vi "DEI_7420_TCP.vi"() -> ()   [LabVIEW 2012]
panel:
  in  "power on exit":bool
  in  "FORCE EXIT":bool
  out "Output Warning":bool
  in  "DEI Current Pulsar":enum32{"Control and Status"}(tab)
  in  "Amp On/Off":bool
  in  "INT TRIG FREQ":i32=7000 min=1000 max=100000 step=1000
  in  "MAIN PULSEWIDTH msec":dbl=1.0 min=0.05 max=5000.0 step=0.001 format="%.3g"
  in  "BIAS PULSEWIDTH msec":dbl=0.025 min=0.0 max=25000.0 step=0.001 format="%.3f"
  in  "BIAS CURRENT (A)":dbl min=0.0 max=5.8 step=0.001 format="%.3f"
  in  "MAIN CURRENT (A)":dbl=10.0 min=0.0 max=15.7 step=0.001 format="%.3g"
  in  "TRIGGER SOURCE":u16(ring)=1 items=["Internal", "External"]
  in  "EXT TRIG TERM (Ohms)":i32=50 min=50 max=10000 step=1
  in  "IP address":string="192.168.0.200"
  out "Int Trig Freq":string
  out "Main Current":string
  out "Main Pulsewidth":string
  out "Bias Current":string
  out "Bias Pulsewidth":string
  out "Ext Trig Term":string
  out "Trigger":string
  in  "Enable Output":bool
  in  "Set Values":bool
  out "Temp Out (C)":dbl
  out "Temp In (C)":dbl
  out "Rear Enable":bool
  out "Keyswitch Enable":bool
  in  "IP timeout ms":i32=1000
  out "Loop Count":i32=13
  in  "EXIT":bool
  # "DEI 7420 Current Pulsar"
  # "DEI\nRESPONSE"
  # "DEI\nCONTROLS"
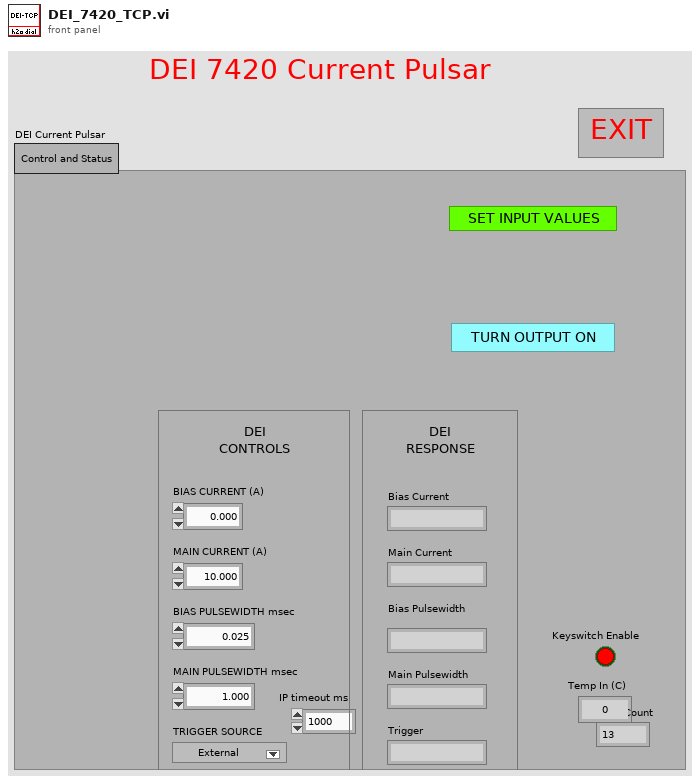
[diagram p1: front panel]
types:
  T1 = enum16{"*IDN?", "BIAS:CURRENT:SETPOINT?", "BIAS:CURRENT:SETPOINT", "FAULT?", "FAULT:CLEAR:ALL", "MAIN:CURRENT:SETPOINT?", "MAIN:CURRENT:SETPOINT", "OUTPUT?", "OUTPUT:DISABLE", "OUTPUT:ENABLE", "*RECALL", "*SAVE", "STATUS:KEYSWITCH?", "STATUS:REAR:ENABLE?", "TEMP:EXHAUST?", "TEMP:IN?", "TRIG?", "TRIG:EXTERNAL", "TRIG:INTERNAL", "TRIG:EXT:TERM?", "TRIG:EXT:TERM", "TRIG:INT:FREQ?", "TRIG:INT:FREQ", "TRIG:INT:BIAS:PULSEWIDTH?", "TRIG:INT:BIAS:PULSEWIDTH", "TRIG:INT:MAIN:PULSEWIDTH?", "TRIG:INT:MAIN:PULSEWIDTH"}
  T2 = enum16{"*IDN?", "BIAS:CURRENT:SETPOINT?", "BIAS:CURRENT:SETPOINT", "FAULT?", "FAULT:CLEAR:ALL", "MAIN:CURRENT:SETPOINT?", "MAIN:CURRENT:SETPOINT", "OUTPUT?", "OUTPUT:DISABLE", "OUTPUT:ENABLE", "*RECALL", "*SAVE", "STATUS:KEYSWITCH?", "STATUS:REAR:ENABLE?", "TEMP:EXHAUST?", "TEMP:IN?", "TRIG?", "TRIG:EXTERNAL", "TRIG:INTERNAL", "TRIG:EXT:TERM?", "TRIG:EXT:TERM", "TRIG:INT:FREQ?", "TRIG:INT:FREQ", "TRIG:INT:BIAS:PULSEWIDTH?", "TRIG:INT:BIAS:PULSEWIDTH", "TRIG:INT:MAIN:PULSEWIDTH?", "TRIG:INT:MAIN:PULSEWIDTH"}[]
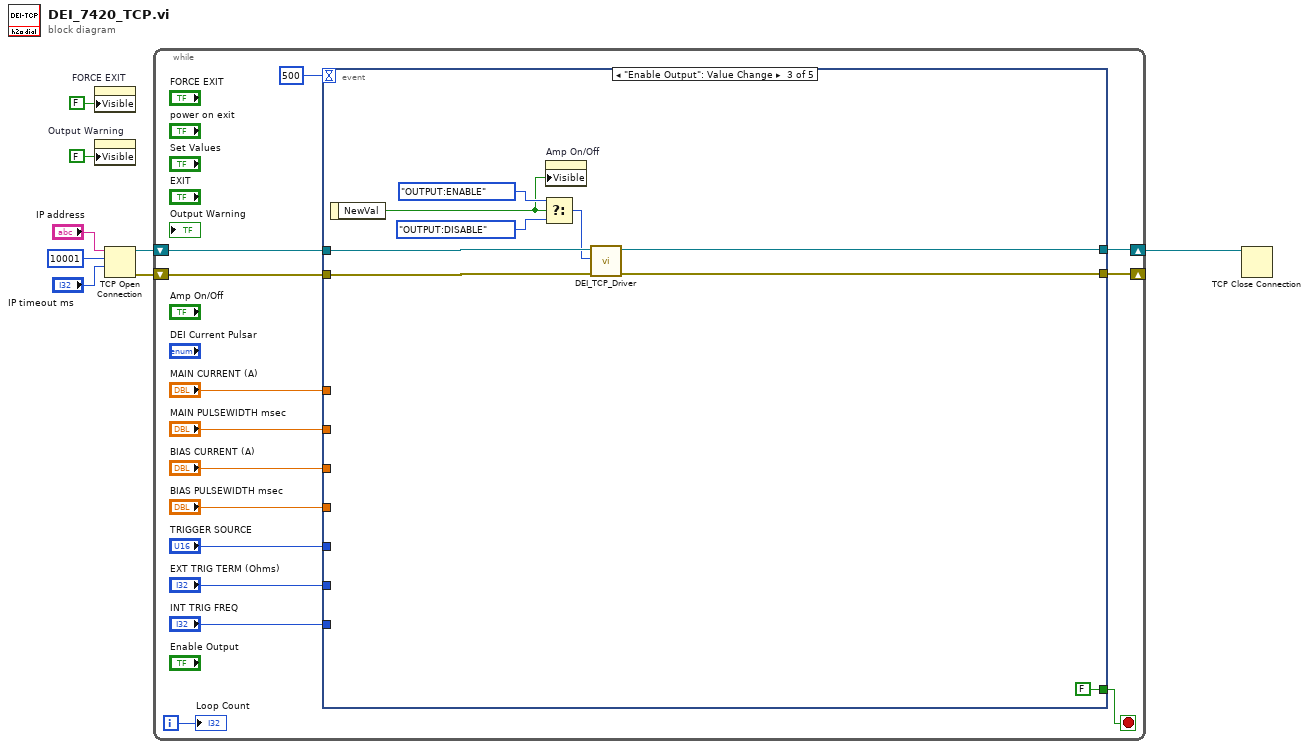
[diagram p0: block diagram]
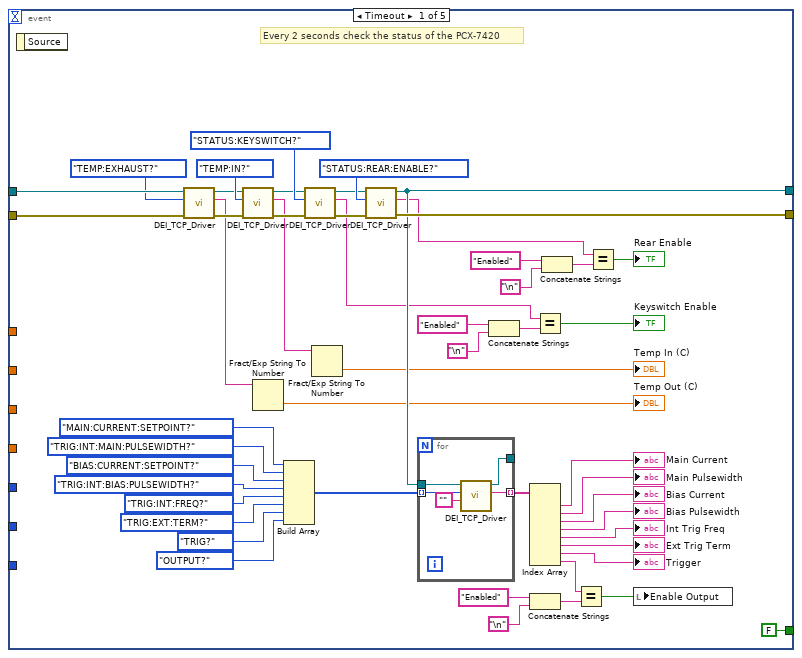
[diagram p2: hidden frame]
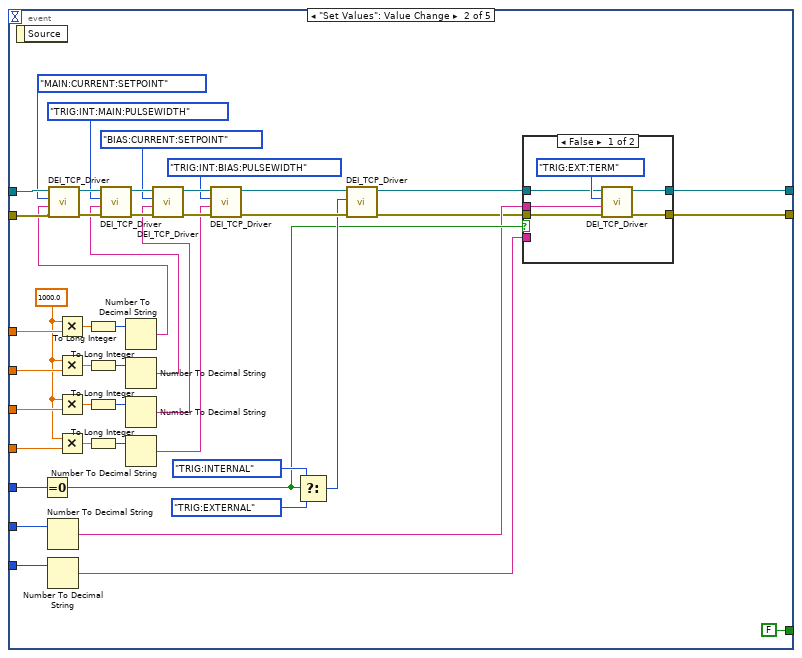
[diagram p3: hidden frame]
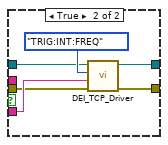
[diagram p4: hidden frame]
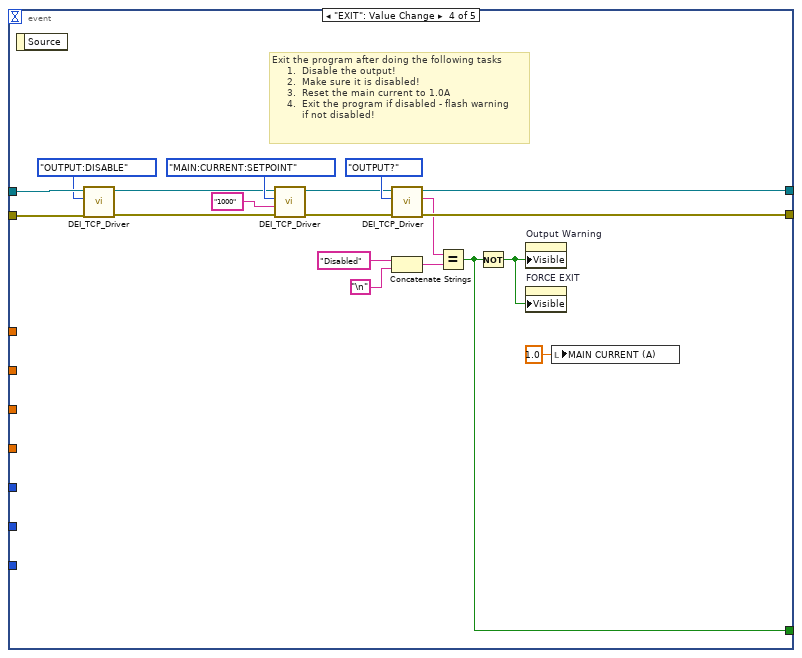
[diagram p5: hidden frame]
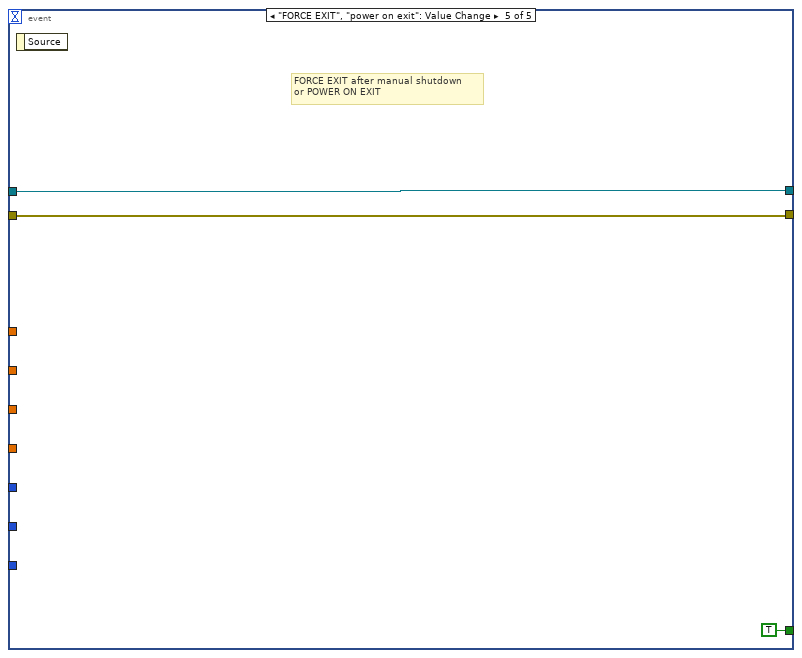
[diagram p6: hidden frame]
diagram:
  n1 = property on="FORCE EXIT" class="Bool"("Visible"=FALSE) -> ()  [unwired: 2 in, 2 out]
  n2 = property on="Output Warning" class="Bool"("Visible"=FALSE) -> ()  [unwired: 2 in, 2 out]
  n3 = TCP Open Connection(address="IP address", remote port or service name=u16 10001, timeout ms (60000)="IP timeout ms") -> (connection ID=w5:refnum<k5>, error out=w8:errorcluster)  [unwired: 2 in]
  n4 = while {
    shift-right: [w20] -> _
    shift-left: w8 -> [w21]
    shift-right: [w11] -> w4
    shift-left: w5 -> [w22]
    i -> [w10]
    stop <- w9 stop-if-true
    n5 = event shown="[2] \"Enable Output\": Value Change" {
      selector: _ -> [_ _ _ _ _]
      dyn-events: _ -> [_ _ _ _ _]
      timeout: 500 -> [_ _ _ _ _]
      tunnel: w22 -> [w71 w123 w143 w163 w165]
      tunnel: w21 -> [w72 w122 w142 w162 w164]
      tunnel: [w69 w115 w139 w161 w165] -> w11
      tunnel: [w70 w114 w140 w160 w164] -> w20
      tunnel: [FALSE FALSE FALSE w152 TRUE] -> w9
      tunnel: "MAIN CURRENT (A)" -> [_ w118 _ _ _]
      tunnel: "MAIN PULSEWIDTH msec" -> [_ w119 _ _ _]
      tunnel: "BIAS CURRENT (A)" -> [_ w120 _ _ _]
      tunnel: "BIAS PULSEWIDTH msec" -> [_ w121 _ _ _]
      tunnel: "TRIGGER SOURCE" -> [_ w116 _ _ _]
      tunnel: "EXT TRIG TERM (Ohms)" -> [_ w117 _ _ _]
      tunnel: "INT TRIG FREQ" -> [_ w113 _ _ _]
      event Timeout {
        # "Every 2 seconds check the status of the PCX-7420"
        n6 = event-data() -> ()  [unwired: 1 in, 1 out]
        n7 = call "DEI_TCP_Driver.vi"("error in"=w72, "DEI COMMANDS"=T1."TEMP:EXHAUST?" ("PCX-7420 COMMANDS"), "connection ID"=w71) -> ("error out"=w63:errorcluster, "read buffer"=w54:string, "connection ID 2"=w66:refnum<k5>)  [unwired: 6 in]
        n8 = call "DEI_TCP_Driver.vi"("error in"=w63, "DEI COMMANDS"=T1."TEMP:IN?" ("PCX-7420 COMMANDS"), "connection ID"=w66) -> ("error out"=w62:errorcluster, "read buffer"=w53:string, "connection ID 2"=w60:refnum<k5>)  [unwired: 6 in]
        n9 = Fract/Exp String To Number(string=w54) -> (number=→"Temp Out (C)":dbl)  [unwired: 3 in, 1 out]
        n10 = Build Array(T1."MAIN:CURRENT:SETPOINT?" ("PCX-7420 COMMANDS"), T1."TRIG:INT:MAIN:PULSEWIDTH?" ("PCX-7420 COMMANDS"), T1."BIAS:CURRENT:SETPOINT?" ("PCX-7420 COMMANDS"), T1."TRIG:INT:BIAS:PULSEWIDTH?" ("PCX-7420 COMMANDS"), T1."TRIG:INT:FREQ?" ("PCX-7420 COMMANDS"), T1."TRIG:EXT:TERM?" ("PCX-7420 COMMANDS"), T1."TRIG?" ("PCX-7420 COMMANDS"), T1."OUTPUT?" ("PCX-7420 COMMANDS")) -> (w42:T2)
        n11 = call "DEI_TCP_Driver.vi"("error in"=w62, "DEI COMMANDS"=T1."STATUS:KEYSWITCH?" ("PCX-7420 COMMANDS"), "connection ID"=w60) -> ("error out"=w61:errorcluster, "read buffer"=w51:string, "connection ID 2"=w59:refnum<k5>)  [unwired: 6 in]
        n12 = Fract/Exp String To Number(string=w53) -> (number=→"Temp In (C)":dbl)  [unwired: 3 in, 1 out]
        n13 = call "DEI_TCP_Driver.vi"("error in"=w61, "DEI COMMANDS"=T1."STATUS:REAR:ENABLE?" ("PCX-7420 COMMANDS"), "connection ID"=w59) -> ("error out"=w70:errorcluster, "read buffer"=w49:string, "connection ID 2"=w69:refnum<k5>)  [unwired: 6 in]
        n14 = for {
          tunnel: w42 -> [w78] mode=indexing
          tunnel: w69 -> [w77]
          tunnel: [w75] -> w41 mode=indexing
          tunnel: [w74] -> _
          n15 = call "DEI_TCP_Driver.vi"("INPUT VALUE"="", "DEI COMMANDS"=w78, "connection ID"=w77) -> ("read buffer"=w75:string, "connection ID 2"=w74:refnum<k5>)  [unwired: 6 in, 1 out]
        }
        n16 = Concatenate Strings("Enabled" ("x"), "\n") -> (w52:string)
        n17 = Index Array(array=w41) -> (element #1=→"Main Current":string, element #2=→"Main Pulsewidth":string, element #3=→"Bias Current":string, element #4=→"Bias Pulsewidth":string, element #5=→"Int Trig Freq":string, element #6=→"Ext Trig Term":string, element #7=→"Trigger":string, element #8=w24:string)  [unwired: 8 in]
        n18 = Concatenate Strings("Enabled" ("x"), "\n") -> (w27:string)
        n19 = Equal?(x=w51, y=w52) -> (x = y?=→"Keyswitch Enable":bool)
        n20 = Concatenate Strings("Enabled" ("x"), "\n") -> (w50:string)
        n21 = Equal?(x=w24, y=w27) -> (x = y?=w26:bool)
        n22 = Equal?(x=w49, y=w50) -> (x = y?=→"Rear Enable":bool)
        n23 = local write "Enable Output"(w26) -> ()
      }
      event "Set Values": Value Change {
        w111 = 1000.0 ("x")
        n24 = event-data() -> ()  [unwired: 1 in, 1 out]
        n25 = Equal To 0?(x=w116) -> (x = 0?=w83:bool)
        n26 = Number To Decimal String(number=w117) -> (decimal integer string=w82:string)  [unwired: 1 in]
        n27 = Number To Decimal String(number=w113) -> (decimal integer string=w81:string)  [unwired: 1 in]
        n28 = Multiply(x=w111, y=w118) -> (x*y=w110:dbl)
        n29 = Multiply(x=w111, y=w119) -> (x*y=w109:dbl)
        n30 = Multiply(x=w111, y=w120) -> (x*y=w108:dbl)
        n31 = Multiply(x=w111, y=w121) -> (x*y=w107:dbl)
        n32 = To Long Integer(number=w110) -> (32bit integer=w103:i32)
        n33 = To Long Integer(number=w109) -> (32bit integer=w104:i32)
        n34 = To Long Integer(number=w108) -> (32bit integer=w105:i32)
        n35 = To Long Integer(number=w107) -> (32bit integer=w106:i32)
        n36 = Number To Decimal String(number=w103) -> (decimal integer string=w101:string)  [unwired: 1 in]
        n37 = call "DEI_TCP_Driver.vi"("error in"=w122, "INPUT VALUE"=w101, "DEI COMMANDS"=T1."MAIN:CURRENT:SETPOINT" ("PCX-7420 COMMANDS"), "connection ID"=w123) -> ("error out"=w97:errorcluster, "connection ID 2"=w100:refnum<k5>)  [unwired: 5 in, 1 out]
        n38 = Number To Decimal String(number=w104) -> (decimal integer string=w93:string)  [unwired: 1 in]
        n39 = call "DEI_TCP_Driver.vi"("error in"=w97, "INPUT VALUE"=w93, "DEI COMMANDS"=T1."TRIG:INT:MAIN:PULSEWIDTH" ("PCX-7420 COMMANDS"), "connection ID"=w100) -> ("error out"=w96:errorcluster, "connection ID 2"=w99:refnum<k5>)  [unwired: 5 in, 1 out]
        n40 = Number To Decimal String(number=w105) -> (decimal integer string=w91:string)  [unwired: 1 in]
        n41 = Number To Decimal String(number=w106) -> (decimal integer string=w89:string)  [unwired: 1 in]
        n42 = call "DEI_TCP_Driver.vi"("error in"=w96, "INPUT VALUE"=w91, "DEI COMMANDS"=T1."BIAS:CURRENT:SETPOINT" ("PCX-7420 COMMANDS"), "connection ID"=w99) -> ("error out"=w95:errorcluster, "connection ID 2"=w98:refnum<k5>)  [unwired: 5 in, 1 out]
        n43 = call "DEI_TCP_Driver.vi"("error in"=w95, "INPUT VALUE"=w89, "DEI COMMANDS"=T1."TRIG:INT:BIAS:PULSEWIDTH" ("PCX-7420 COMMANDS"), "connection ID"=w98) -> ("error out"=w86:errorcluster, "connection ID 2"=w85:refnum<k5>)  [unwired: 5 in, 1 out]
        n44 = Select(t=T1."TRIG:INTERNAL" ("PCX-7420 COMMANDS"), s=w83, f=T1."TRIG:EXTERNAL" ("PCX-7420 COMMANDS")) -> (s? t:f=w84:T1)
        n45 = call "DEI_TCP_Driver.vi"("error in"=w86, "DEI COMMANDS"=w84, "connection ID"=w85) -> ("error out"=w79:errorcluster, "connection ID 2"=w80:refnum<k5>)  [unwired: 6 in, 1 out]
        n46 = case shown="False" w83 {
          tunnel: [w129 w135] -> w115
          tunnel: [w128 w134] -> w114
          tunnel: w82 -> [w127 _]
          tunnel: w81 -> [_ w132]
          tunnel: w80 -> [w124 w131]
          tunnel: w79 -> [w125 w130]
          frame False {
            n47 = call "DEI_TCP_Driver.vi"("error in"=w125, "INPUT VALUE"=w127, "DEI COMMANDS"=T1."TRIG:EXT:TERM" ("PCX-7420 COMMANDS"), "connection ID"=w124) -> ("error out"=w128:errorcluster, "connection ID 2"=w129:refnum<k5>)  [unwired: 5 in, 1 out]
          }
          frame True {
            n48 = call "DEI_TCP_Driver.vi"("error in"=w130, "INPUT VALUE"=w132, "DEI COMMANDS"=T1."TRIG:INT:FREQ" ("PCX-7420 COMMANDS"), "connection ID"=w131) -> ("error out"=w134:errorcluster, "connection ID 2"=w135:refnum<k5>)  [unwired: 5 in, 1 out]
          }
        }
      }
      event "Enable Output": Value Change {
        n49 = event-data() -> ("NewVal"=w136:bool)  [unwired: 1 in]
        n50 = Select(t=T1."OUTPUT:ENABLE" ("PCX-7420 COMMANDS"), s=w136, f=T1."OUTPUT:DISABLE" ("PCX-7420 COMMANDS")) -> (s? t:f=w141:T1)
        n51 = property on="Amp On/Off" class="Bool"("Visible"=w136) -> ()  [unwired: 2 in, 2 out]
        n52 = call "DEI_TCP_Driver.vi"("error in"=w142, "DEI COMMANDS"=w141, "connection ID"=w143) -> ("error out"=w140:errorcluster, "connection ID 2"=w139:refnum<k5>)  [unwired: 6 in, 1 out]
      }
      event "EXIT": Value Change {
        # "Exit the program after doing the following tasks\n     1.  Disable the output!\n     2.  Make sure it is disabled!\n     3.  Reset the main current to 1.0A\n     4.  Exit the program if disabled - flash warning\n          if not disabled!"
        n53 = event-data() -> ()  [unwired: 1 in, 1 out]
        n54 = call "DEI_TCP_Driver.vi"("error in"=w162, "DEI COMMANDS"=T1."OUTPUT:DISABLE" ("PCX-7420 COMMANDS"), "connection ID"=w163) -> ("error out"=w148:errorcluster, "connection ID 2"=w149:refnum<k5>)  [unwired: 6 in, 1 out]
        n55 = call "DEI_TCP_Driver.vi"("error in"=w148, "INPUT VALUE"="1000", "DEI COMMANDS"=T1."MAIN:CURRENT:SETPOINT" ("PCX-7420 COMMANDS"), "connection ID"=w149) -> ("error out"=w146:errorcluster, "connection ID 2"=w147:refnum<k5>)  [unwired: 5 in, 1 out]
        n56 = call "DEI_TCP_Driver.vi"("error in"=w146, "DEI COMMANDS"=T1."OUTPUT?" ("PCX-7420 COMMANDS"), "connection ID"=w147) -> ("error out"=w160:errorcluster, "read buffer"=w154:string, "connection ID 2"=w161:refnum<k5>)  [unwired: 6 in]
        n57 = Concatenate Strings("Disabled" ("x"), "\n") -> (w155:string)
        n58 = Equal?(x=w154, y=w155) -> (x = y?=w152:bool)
        n59 = Not(x=w152) -> (.not. x?=w153:bool)
        n60 = property on="Output Warning" class="Bool"("Visible"=w153) -> ()  [unwired: 2 in, 2 out]
        n61 = property on="FORCE EXIT" class="Bool"("Visible"=w153) -> ()  [unwired: 2 in, 2 out]
        n62 = local write "MAIN CURRENT (A)"(1.0 ("MAIN CURRENT (A)")) -> ()
      }
      event "FORCE EXIT", "power on exit": Value Change {
        # "FORCE EXIT after manual shutdown\nor POWER ON EXIT"
        n63 = event-data() -> ()  [unwired: 1 in, 1 out]
      }
    }
    "Loop Count" <- w10
  }
  n64 = TCP Close Connection(connection ID=w4) -> ()  [unwired: 2 in, 2 out]
